vi "MoveDown.vi"(0 "Grids In":i32[][](array[numeric])) -> (1 "Grids Out":i32[][](array[numeric]), 2 "Score":i32, 3 "Moved?":bool)   [LabVIEW 2018]
doc: "Move grids down."
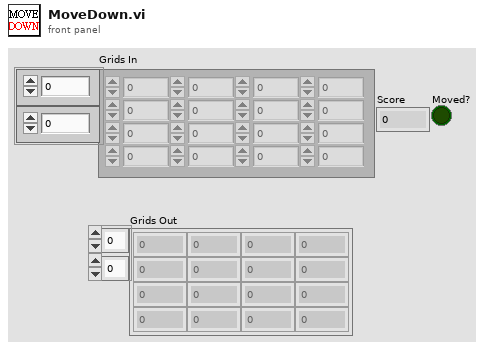
[diagram p1: front panel]
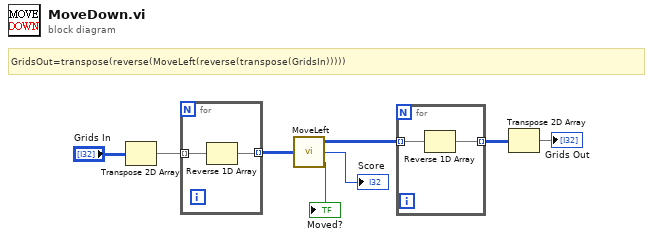
[diagram p0: block diagram]
diagram:
  # "GridsOut=transpose(reverse(MoveLeft(reverse(transpose(GridsIn)))))"
  n1 = Transpose 2D Array(2D array="Grids In") -> (transposed array=w7:i32[][])
  n2 = for {
    tunnel: w7 -> [w10] mode=indexing
    tunnel: [w9] -> w6 mode=indexing
    n3 = Reverse 1D Array(array=w10) -> (reversed array=w9:i32[])
  }
  n4 = call "MoveLeft.vi"("Grids In"=w6) -> ("Grid Out"=w5:i32[][], "Score"=→"Score":i32, "Moved?"=→"Moved?":bool)
  n5 = for {
    tunnel: w5 -> [w12] mode=indexing
    tunnel: [w11] -> w4 mode=indexing
    n6 = Reverse 1D Array(array=w12) -> (reversed array=w11:i32[])
  }
  n7 = Transpose 2D Array(2D array=w4) -> (transposed array=→"Grids Out":i32[][])
